vi "NumberGen.vi"() -> ()   [LabVIEW 2019]
panel:
  out "Waveform Chart":dbl[][](graph)
  in  "x1":dbl
  in  "x2":dbl
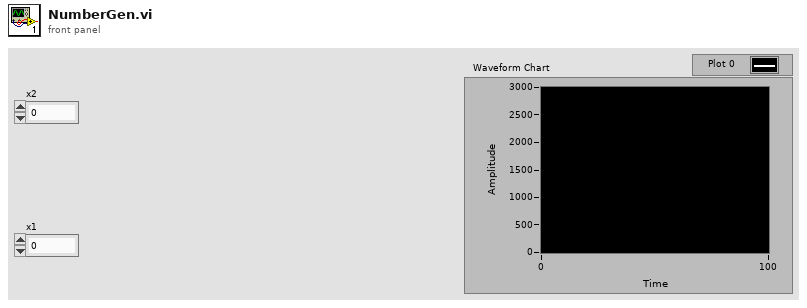
[diagram p1: front panel]
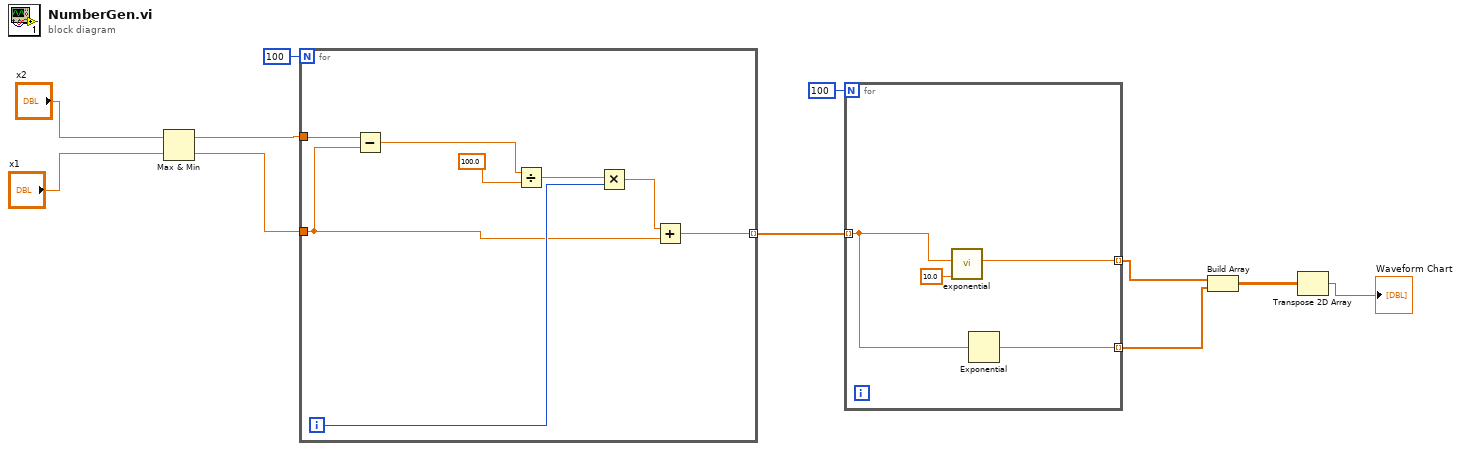
[diagram p0: block diagram]
diagram:
  n1 = Max & Min(x="x2", y="x1") -> (max(x,y)=w6:dbl, min(x,y)=w5:dbl)
  n2 = for {
    N: 100 -> [_]
    tunnel: w5 -> [w14]
    tunnel: w6 -> [w18]
    tunnel: [w12] -> w10 mode=indexing
    i -> [w16]
    n3 = Subtract(x=w18, y=w14) -> (x-y=w17:dbl)
    n4 = Divide(x=w17, y=100.0) -> (x/y=w15:dbl)
    n5 = Multiply(x=w15, y=w16) -> (x*y=w13:dbl)
    n6 = Add(x=w13, y=w14) -> (x+y=w12:dbl)
  }
  n7 = for {
    N: 100 -> [_]
    tunnel: w10 -> [w21] mode=indexing
    tunnel: [w22] -> w4 mode=indexing
    tunnel: [w20] -> w3 mode=indexing
    n8 = call "exponential.vi"("n"=10.0, "x"=w21) -> ("exp(x)"=w22:dbl)  [unwired: 9 in]
    n9 = Exponential(1:w21) -> (0:w20:dbl)
  }
  n10 = Build Array(w4, w3) -> (w2:dbl[][])
  n11 = Transpose 2D Array(2D array=w2) -> (transposed array=→"Waveform Chart":dbl[][])
